vi "DAQtetris.vi"() -> ()   [LabVIEW 2018]
uses:
  <vilib>/Analysis/3filter.llb/Filter Passband Type.ctl
  <vilib>/Instr/_visa.llb/VISA Configure Serial Port (Instr).vi
  <vilib>/Analysis/3filter.llb/Butterworth Filter (DBL).vi
  <vilib>/Utility/file.llb/Write Delimited Spreadsheet (I64).vi
  <vilib>/Analysis/NI_AALBase.lvlib
panel:
  in  "Cancel Button":bool=TRUE
  out "error out":errorcluster
  out "stop 2":bool=TRUE
  in  "error in (no error)":errorcluster
  in  "Python version":string="3.6"
  out "AI2 2":i16(graph)
  out "AI1 2":i16(graph)
  out "AI0 2":i16(graph)
  in  "y 3":i16=8
  in  "y 2":i16=4
  in  "y":i16=7
  out "Up":bool
  out "Right":bool
  out "Left":bool
  in  "TR":dbl(slide)=2.5718194254445967e-05 scale=0.0..0.0001 scale format="%#_9g"
  in  "TT":dbl(slide)=2.633744855967078e-05 scale=0.0..0.0001 scale format="%#_9g"
  in  "TL":dbl(slide)=4.78796169630643e-05 scale=0.0..0.0001 scale format="%#_9g"
  in  "Rang 3":dbl(knob)=1000.0 scale=0.0..2000.0
  in  "Rang 2":dbl(knob)=1000.0 scale=0.0..2000.0
  in  "Rang 1":dbl(knob)=1000.0 scale=0.0..2000.0
  in  "File name":string="data111"
  in  "Record Button":bool
  out "Data Size":i32=4943
  out "Time left":u32
  in  "Time length(ms)":i32=100000
  in  "Timer":bool
  out "appended array":u16[][](array[numeric])
  out "Loop Time":u32
  in  "baud rate (9600)":u32=256000
  out "AI2":u16(graph)=19
  out "AI1":u16(graph)
  in  "Command":string="\u0000\u0000\u0006\u0004"
  in  "Disconnect":bool
  in  "Connect":bool
  out "AI0":u16(graph)=51
  in  "Send Command":bool
  in  "stop":bool
  out "read buffer":string
  in  "VISA resource name":refnum<visa-resource-name>="COM3"
  # "meDAQ v1.0\nXiangpeng"
  # "Wireless DAQ for Wearable Device"
  # "L"
  # "Display Scale"
  # "Initialization"
  # "Data Recording"
  # "T"
  # "Advanced Bluetooth Operation"
  # "R"
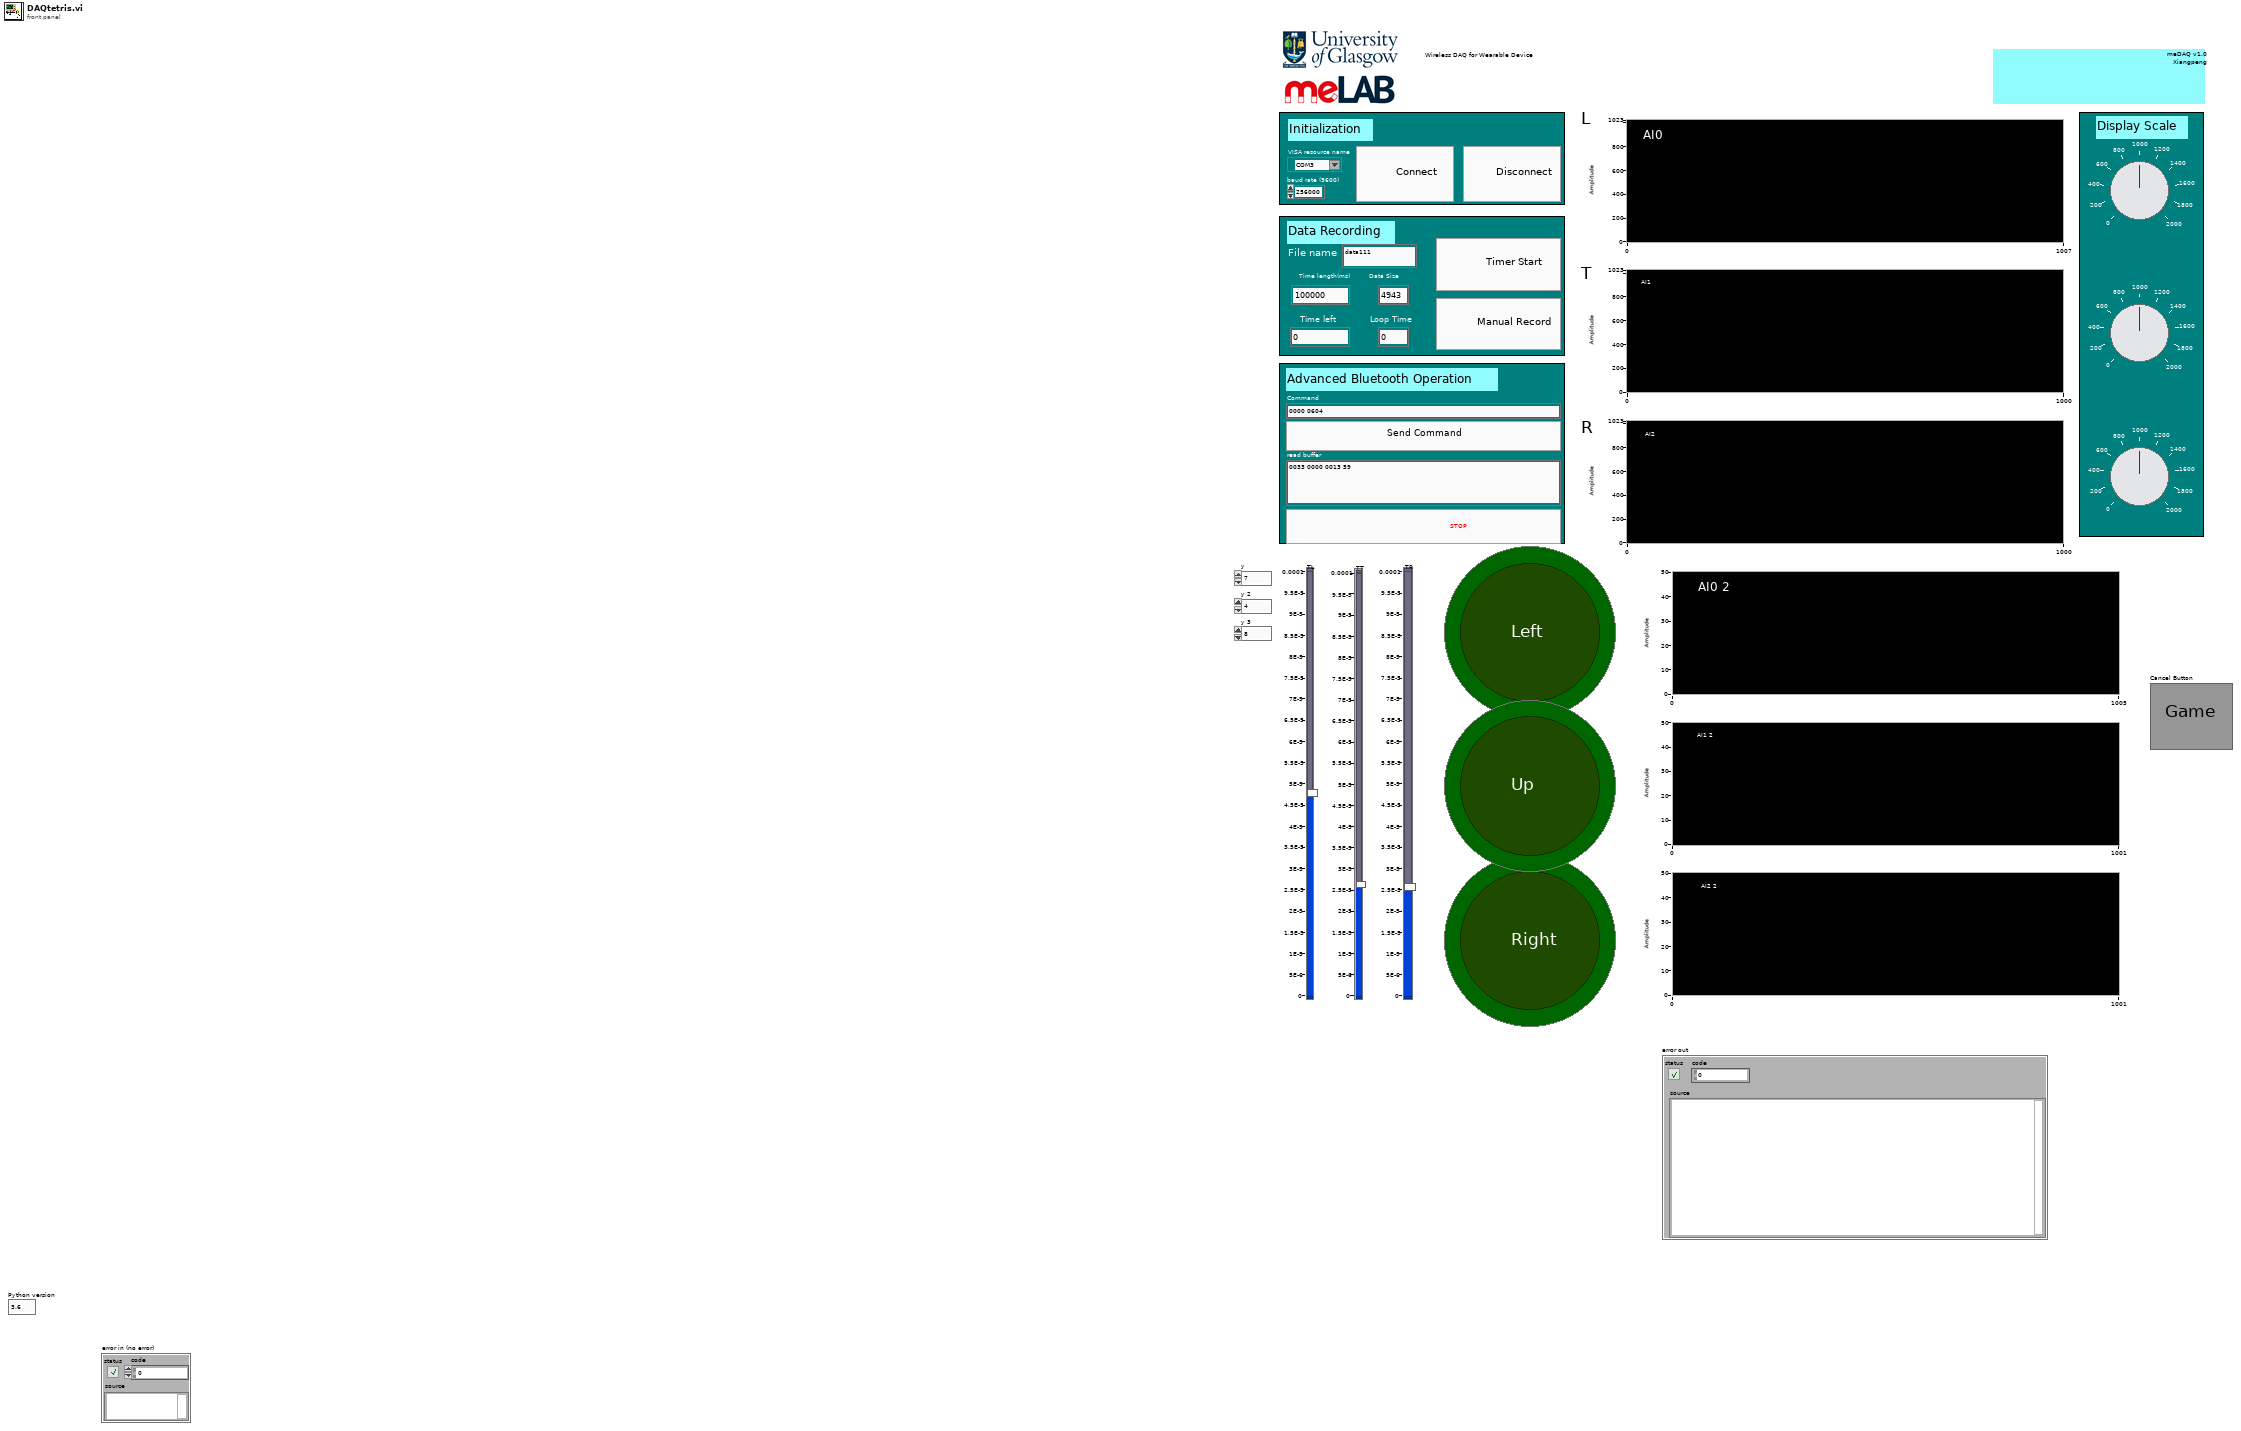
[diagram p1: front panel]
types:
  T1 = typedef "Sound Output Task ID.ctl" = u32
  T2 = typedef "NI_AALBase.lvlib/Filter Passband Type.ctl" = enum32{"Lowpass", "Highpass", "Bandpass", "Bandstop"}
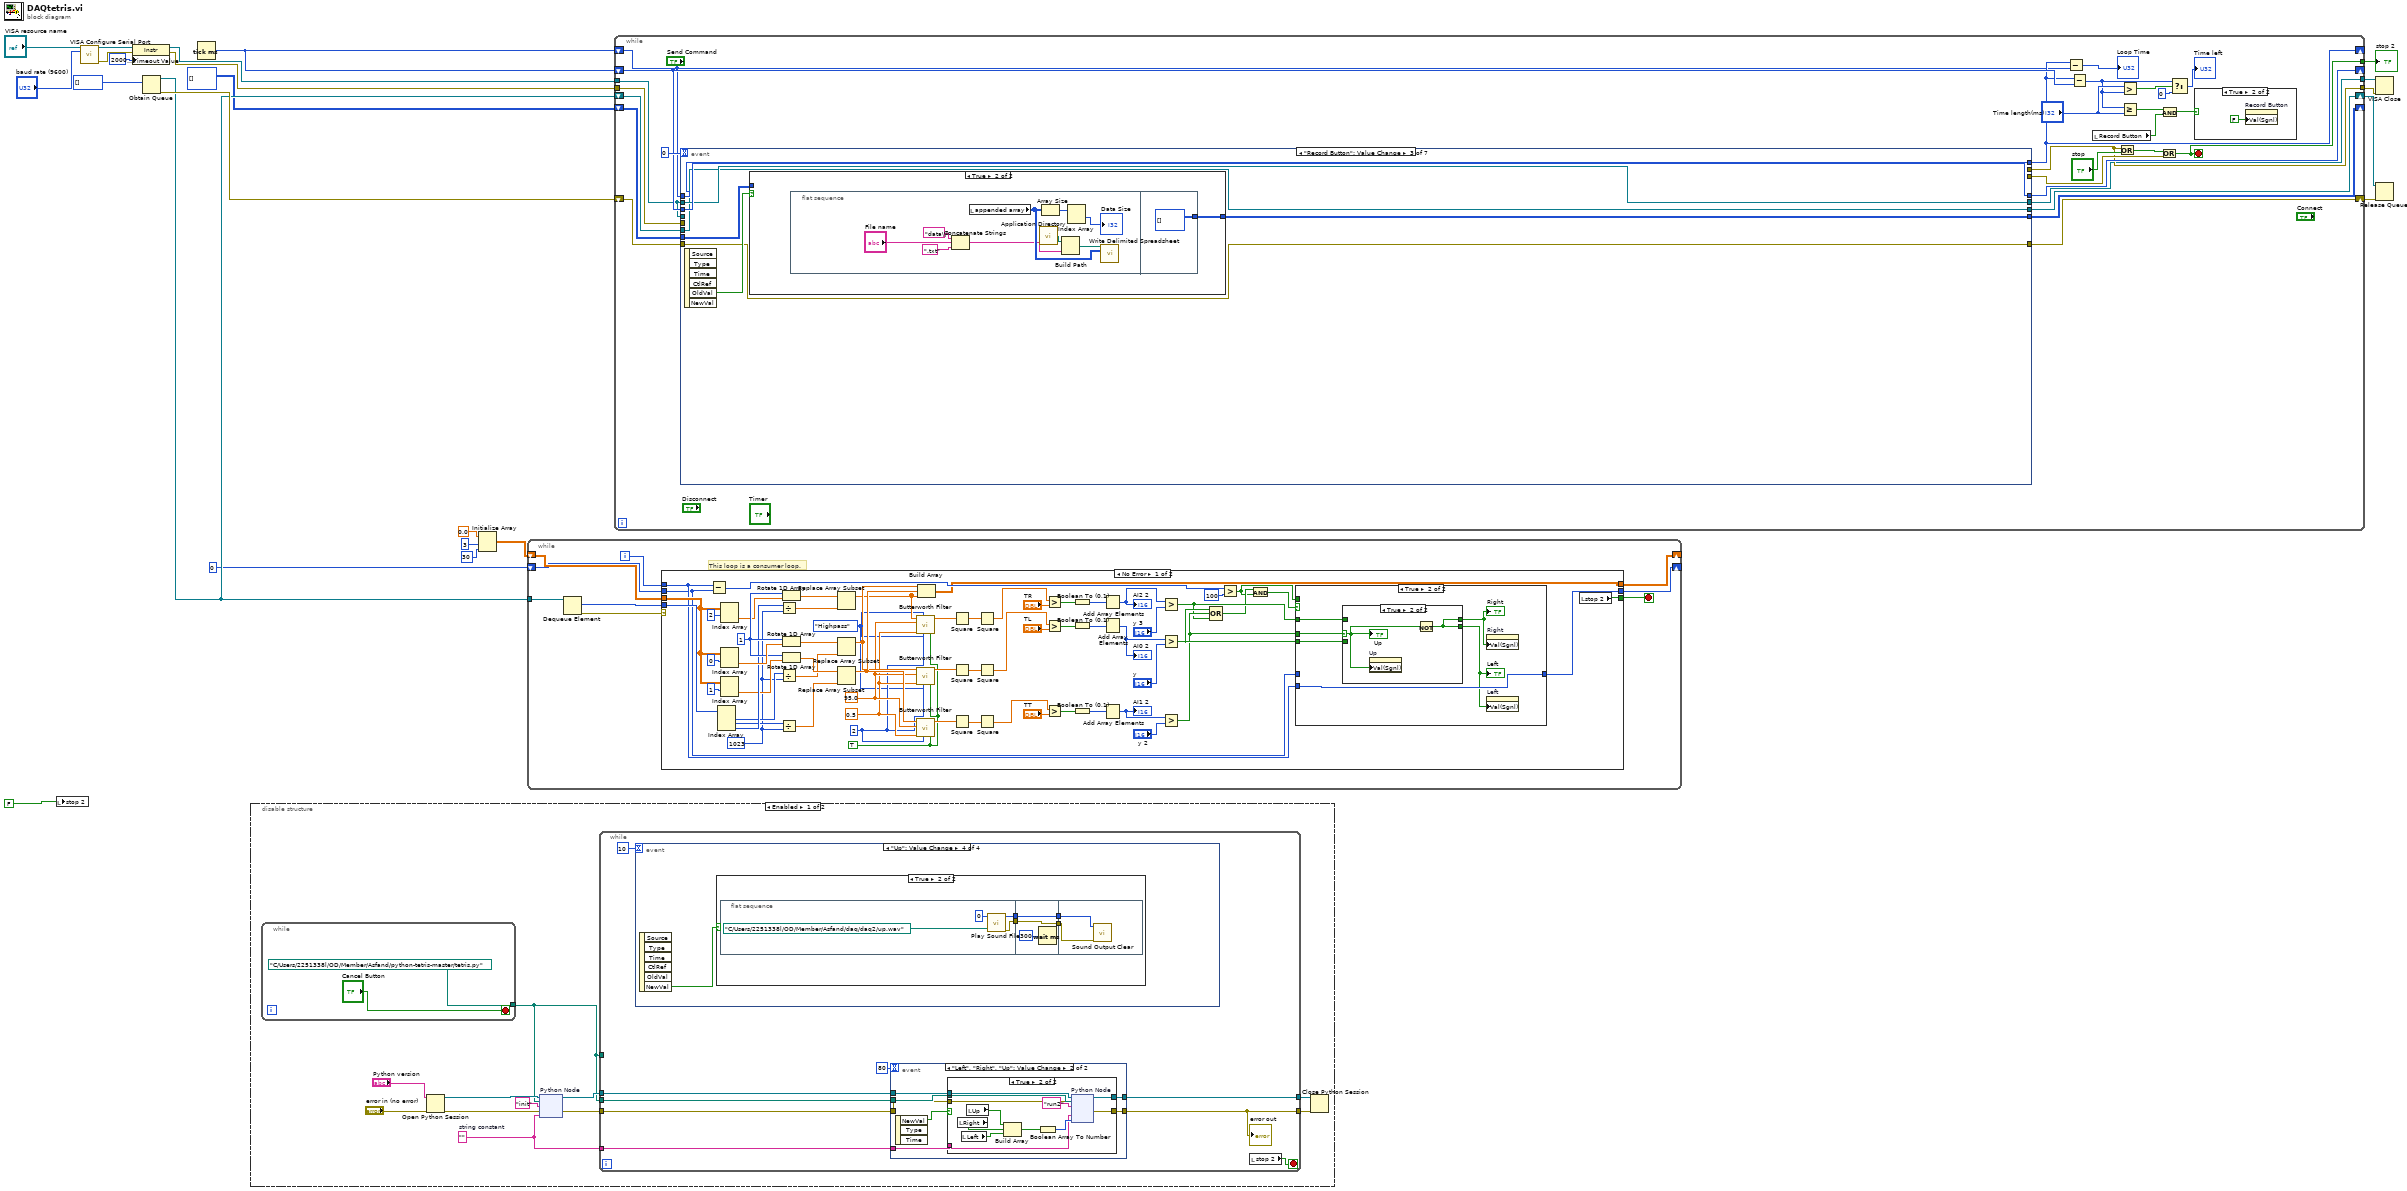
[diagram p0: block diagram]
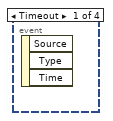
[diagram p2: hidden frame]
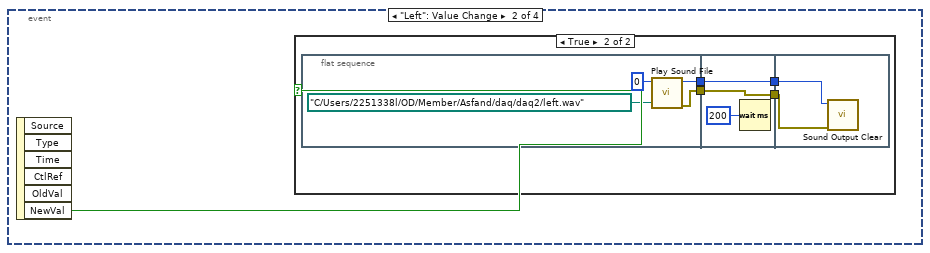
[diagram p3: hidden frame]
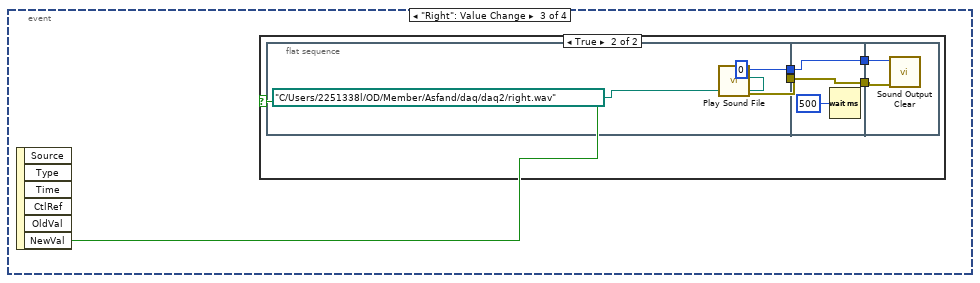
[diagram p5: hidden frame]
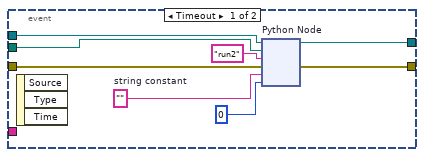
[diagram p8: hidden frame]
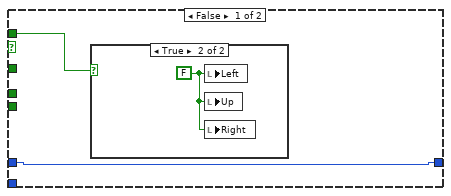
[diagram p11: hidden frame]
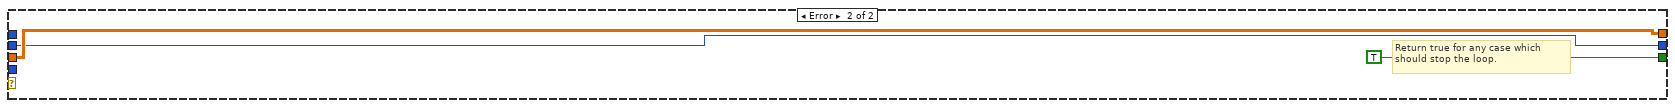
[diagram p14: hidden frame]
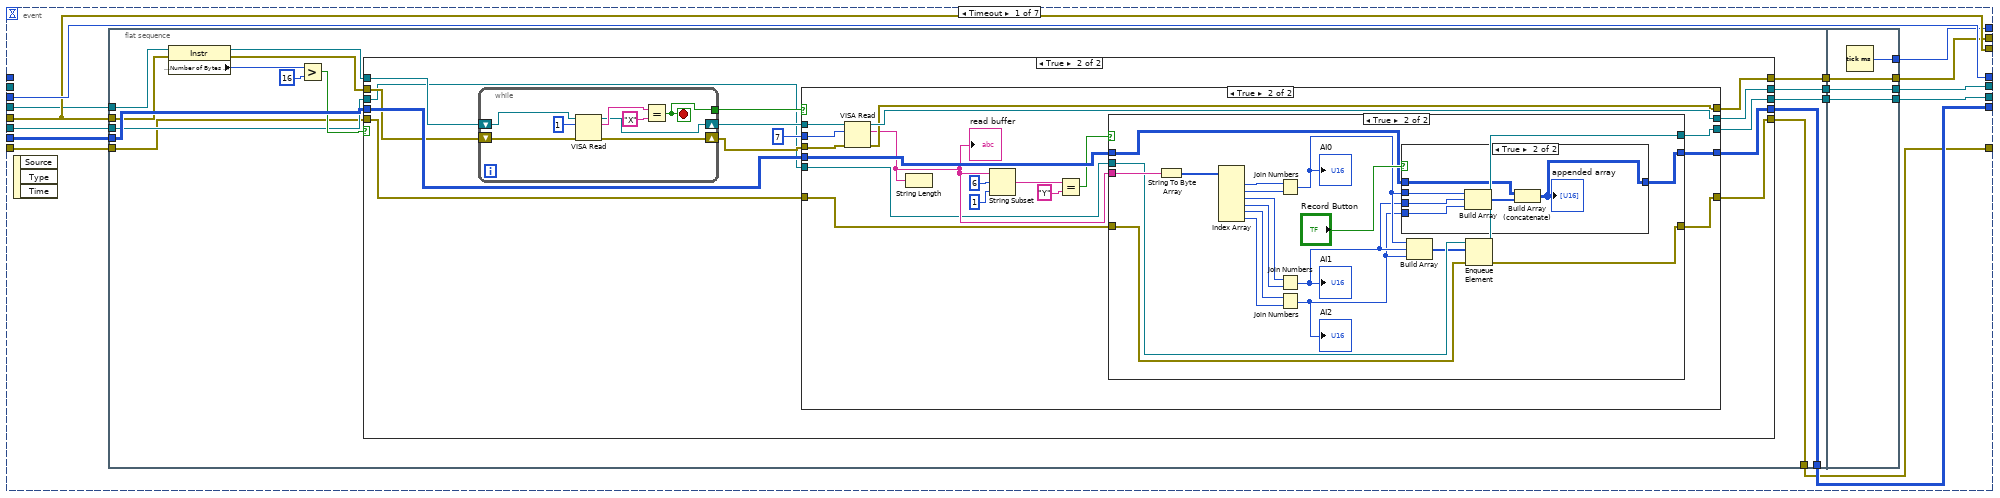
[diagram p16: hidden frame]
diagram:
  n1 = local write "stop 2"(FALSE ("stop 2")) -> ()
  n2 = call-poly "VISA Configure Serial Port"("VISA resource name"="VISA resource name", "baud rate (9600)"="baud rate (9600)") -> ("VISA resource name out"=w17:refnum<visa-resource-name>, "error out"=w16:errorcluster)  [unwired: 12 in]
  n3 = property class="Instr"(reference=w17, error in=w16, "General Settings:Timeout Value"=u32 2000) -> (reference out=w14:refnum<visa-resource-name>, error out=w15:errorcluster)
  n4 = Obtain Queue(element data type=u16[] []) -> (queue out=w10:refnum<queue>, error out=w13:errorcluster)  [unwired: 4 in, 1 out]
  n5 = Tick Count (ms)() -> (millisecond timer value=w19:u32)
  n6 = disable-structure shown="Enabled" {
    frame Enabled {
      w25 = ""  # string constant
      n7 = while {
        tunnel: [path "C:/Users/2251338l/OD/Member/Asfand/python-tetris-master/tetris.py" ("module path")] -> w24
        stop <- "Cancel Button" stop-if-true
      }
      n8 = Open Python Session(python version="Python version", 3:"error in (no error)") -> (session out=w31:refnum<k35>, error out=w30:errorcluster)  [unwired: 1 in]
      n9 = node "Python Node"(w31, w24, "init" ("function name"), w30, w25) -> (w27:refnum<k35>, w26:errorcluster)  [unwired: 1 in, 2 out]
      n10 = while {
        tunnel: [w37] -> w29
        tunnel: [w41] -> w28
        tunnel: w27 -> [w44]
        tunnel: w26 -> [w43]
        tunnel: w24 -> [w42]
        tunnel: w25 -> [w38]
        tunnel: w24 -> [_]
        stop <- w40 stop-if-true
        n11 = event shown="[3] \"Up\": Value Change" {
          selector: _ -> [_ _ _ _]
          dyn-events: _ -> [_ _ _ _]
          timeout: 10 -> [_ _ _ _]
          event Timeout {
            n12 = event-data() -> ()  [unwired: 1 in, 3 out]
          }
          event "Left": Value Change {
            n13 = event-data() -> ("NewVal"=w46:bool)  [unwired: 1 in, 5 out]
            n14 = case shown="True" w46 {
              frame False {
              }
              frame True {
                n15 = flat-sequence {
                  tunnel: [w54] -> w50
                  tunnel: [w51] -> w47
                  tunnel: w50 -> [w57]
                  tunnel: [w57] -> w49
                  tunnel: [w55] -> w48
                  tunnel: w47 -> [w55]
                  tunnel: w49 -> [w58]
                  tunnel: w48 -> [w59]
                  frame #0 {
                    n16 = call <vilib>:"Play Sound File.vi"("path"=path "C:/Users/2251338l/OD/Member/Asfand/daq/daq2/left.wav" ("Sound File Path"), "device ID"=u32 0) -> ("error out"=w51:errorcluster, "task ID"=w54:T1)  [unwired: 8 in]
                  }
                  frame #1 {
                    n17 = Wait (ms)(milliseconds to wait=u32 200) -> ()  [unwired: 1 out]
                  }
                  frame #2 {
                    n18 = call <vilib>:"Sound Output Clear.vi"("error in (no error)"=w59, "task ID"=w58) -> ()  [unwired: 9 in, 1 out]
                  }
                }
              }
            }
          }
          event "Right": Value Change {
            n19 = event-data() -> ("NewVal"=w60:bool)  [unwired: 1 in, 5 out]
            n20 = case shown="True" w60 {
              frame False {
              }
              frame True {
                n21 = flat-sequence {
                  tunnel: [w68] -> w64
                  tunnel: [w66] -> w63
                  tunnel: w64 -> [w69]
                  tunnel: [w70] -> w62
                  tunnel: w63 -> [w70]
                  tunnel: [w69] -> w61
                  tunnel: w62 -> [w73]
                  tunnel: w61 -> [w72]
                  frame #0 {
                    n22 = call <vilib>:"Play Sound File.vi"("path"=path "C:/Users/2251338l/OD/Member/Asfand/daq/daq2/right.wav" ("Sound File Path"), "device ID"=u32 0) -> ("error out"=w66:errorcluster, "task ID"=w68:T1)  [unwired: 8 in]
                  }
                  frame #1 {
                    n23 = Wait (ms)(milliseconds to wait=u32 500) -> ()  [unwired: 1 out]
                  }
                  frame #2 {
                    n24 = call <vilib>:"Sound Output Clear.vi"("error in (no error)"=w73, "task ID"=w72) -> ()  [unwired: 9 in, 1 out]
                  }
                }
              }
            }
          }
          event "Up": Value Change {
            n25 = event-data() -> ("NewVal"=w74:bool)  [unwired: 1 in, 5 out]
            n26 = case shown="True" w74 {
              frame False {
              }
              frame True {
                n27 = flat-sequence {
                  tunnel: [w82] -> w78
                  tunnel: [w80] -> w77
                  tunnel: w78 -> [w85]
                  tunnel: [w85] -> w76
                  tunnel: [w83] -> w75
                  tunnel: w77 -> [w83]
                  tunnel: w76 -> [w86]
                  tunnel: w75 -> [w87]
                  frame #0 {
                    n28 = call <vilib>:"Play Sound File.vi"("path"=path "C:/Users/2251338l/OD/Member/Asfand/daq/daq2/up.wav" ("Sound File Path"), "device ID"=u32 0) -> ("error out"=w80:errorcluster, "task ID"=w82:T1)  [unwired: 8 in]
                  }
                  frame #1 {
                    n29 = Wait (ms)(milliseconds to wait=u32 300) -> ()  [unwired: 1 out]
                  }
                  frame #2 {
                    n30 = call <vilib>:"Sound Output Clear.vi"("error in (no error)"=w87, "task ID"=w86) -> ()  [unwired: 9 in, 1 out]
                  }
                }
              }
            }
          }
        }
        n31 = event shown="[1] \"Left\", \"Right\", \"Up\": Value Change" {
          selector: _ -> [_ _]
          dyn-events: _ -> [_ _]
          timeout: 80 -> [_ _]
          tunnel: w44 -> [w95 w98]
          tunnel: w43 -> [w93 w99]
          tunnel: w42 -> [w91 w102]
          tunnel: [w90 w101] -> w37
          tunnel: [w89 w100] -> w41
          tunnel: w38 -> [_ w97]
          event Timeout {
            w92 = ""  # string constant
            n32 = event-data() -> ()  [unwired: 1 in, 3 out]
            n33 = node "Python Node"(w95, w91, "run2" ("function name"), w93, w92, u32 0 ("device ID")) -> (w90:refnum<k35>, w89:errorcluster)  [unwired: 2 in, 2 out]
          }
          event "Left", "Right", "Up": Value Change {
            n34 = event-data() -> ("NewVal"=w96:bool)  [unwired: 1 in, 2 out]
            n35 = case shown="True" w96 {
              tunnel: w102 -> [_ w111]
              tunnel: [w104 w109] -> w101
              tunnel: [w103 w108] -> w100
              tunnel: w99 -> [w103 w107]
              tunnel: w98 -> [w104 w106]
              tunnel: w97 -> [_ w105]
              frame False {
              }
              frame True {
                n36 = local read "Right"() -> (w114:bool)
                n37 = local read "Left"() -> (w113:bool)
                n38 = local read "Up"() -> (w115:bool)
                n39 = Build Array(w115, w114, w113) -> (w112:bool[])
                n40 = Boolean Array To Number(Boolean array=w112) -> (number=w116:u32)
                n41 = node "Python Node"(w106, w111, "run2" ("function name"), w107, w105, w116) -> (w109:refnum<k35>, w108:errorcluster)  [unwired: 2 in, 2 out]
              }
            }
          }
        }
        "error out" <- w41
        n42 = local read "stop 2"() -> (w40:bool)
      }
      n43 = Close Python Session(session in=w29, error in=w28) -> ()  [unwired: 1 out]
    }
    frame Disabled {
    }
  }
  n44 = Initialize Array(0.0, 3 ("dimension size"), 30 ("dimension size")) -> (w4:dbl[][])
  n45 = while {
    tunnel: w10 -> [w125]
    shift-right: [w120] -> _
    shift-left: w4 -> [w121]
    shift-right: [w119] -> _
    shift-left: 0 -> [w117]
    i -> [w118]
    stop <- w122 stop-if-true
    # "This loop is a consumer loop."
    n46 = Dequeue Element(queue=w125) -> (element=w123:u16[], error out=w124:errorcluster)  [unwired: 2 in, 2 out]
    n47 = case shown="No Error" w124 {
      tunnel: w123 -> [w187 _]
      tunnel: [w126 TRUE] -> w122
      tunnel: w121 -> [w181 w204]
      tunnel: [w138 w204] -> w120
      tunnel: [w146 w203] -> w119
      tunnel: w118 -> [w145 _]
      tunnel: w117 -> [w144 w203]
      frame No Error {
        w128 = TRUE ("init/cont (init:F)")
        w131 = 95.0 ("sampling freq: fs")
        w129 = 2 ("order")
        w130 = 0.5 ("low cutoff freq: fl")
        w127 = Filter_Passband_Type."Highpass" ("filter type")
        w157 = u16 1023 ("y")
        w186 = 1 ("n")
        n48 = Subtract(x=w145, y=w144) -> (x-y=w143:i32)
        n49 = Index Array(array=w187) -> (element #1=w161:u16, element #2=w182:u16, element #3=w183:u16)  [unwired: 3 in]
        n50 = Index Array(array=w181, index (row)=2 ("index (col)")) -> (element=w179:dbl[])  [unwired: 1 in]
        n51 = Index Array(array=w181, index (row)=0 ("disabled index (col)")) -> (element=w189:dbl[])  [unwired: 1 in]
        n52 = Index Array(array=w181, index (row)=1 ("index (col)")) -> (element=w180:dbl[])  [unwired: 1 in]
        n53 = Divide(x=w183, y=w157) -> (x/y=w158:dbl)
        n54 = Divide(x=w161, y=w157) -> (x/y=w160:dbl)
        n55 = Divide(x=w182, y=w157) -> (x/y=w159:dbl)
        n56 = Rotate 1D Array(1:w179, 2:w186) -> (0:w184:dbl[])
        n57 = Rotate 1D Array(1:w189, 2:w186) -> (0:w188:dbl[])
        n58 = Rotate 1D Array(1:w180, 2:w186) -> (0:w185:dbl[])
        n59 = Replace Array Subset(array=w184, new element=w158) -> (w133:dbl[])  [unwired: 1 in]
        n60 = Replace Array Subset(array=w188, new element=w160) -> (w135:dbl[])  [unwired: 1 in]
        n61 = Replace Array Subset(array=w185, new element=w159) -> (w137:dbl[])  [unwired: 1 in]
        n62 = call-poly <vilib>:"Butterworth Filter.vi"("init/cont (init:F)"=w128, "order"=w129, "filter type"=w127, "low cutoff freq: fl"=w130, "sampling freq: fs"=w131, "X"=w133) -> ("Filtered X"=w132:dbl[])  [unwired: 2 in, 1 out]
        n63 = call-poly <vilib>:"Butterworth Filter.vi"("init/cont (init:F)"=w128, "order"=w129, "filter type"=w127, "low cutoff freq: fl"=w130, "sampling freq: fs"=w131, "X"=w135) -> ("Filtered X"=w134:dbl[])  [unwired: 2 in, 1 out]
        n64 = call-poly <vilib>:"Butterworth Filter.vi"("init/cont (init:F)"=w128, "order"=w129, "filter type"=w127, "low cutoff freq: fl"=w130, "sampling freq: fs"=w131, "X"=w137) -> ("Filtered X"=w136:dbl[])  [unwired: 2 in, 1 out]
        n65 = Build Array(w135, w137, w133) -> (w138:dbl[][])
        n66 = Square(x=w132) -> (x^2=w156:dbl[])
        n67 = Square(x=w134) -> (x^2=w154:dbl[])
        n68 = Square(x=w136) -> (x^2=w155:dbl[])
        n69 = Square(x=w156) -> (x^2=w171:dbl[])
        n70 = Square(x=w154) -> (x^2=w175:dbl[])
        n71 = Square(x=w155) -> (x^2=w170:dbl[])
        n72 = Greater?(x=w171, y="TR") -> (0:w162:bool[])
        n73 = Greater?(x=w175, y="TL") -> (0:w169:bool[])
        n74 = Greater?(x=w170, y="TT") -> (0:w165:bool[])
        n75 = Boolean To (0,1)(Boolean=w162) -> (0, 1=w164:i16[])
        n76 = Boolean To (0,1)(Boolean=w169) -> (0, 1=w168:i16[])
        n77 = Boolean To (0,1)(Boolean=w165) -> (0, 1=w166:i16[])
        n78 = Add Array Elements(numeric array=w164) -> (sum=w153:i16)
        "AI2 2" <- w153
        n79 = Add Array Elements(numeric array=w168) -> (sum=w151:i16)
        "AI0 2" <- w151
        n80 = Add Array Elements(numeric array=w166) -> (sum=w152:i16)
        "AI1 2" <- w152
        n81 = Greater?(x=w153, y="y 3") -> (0:w148:bool)
        n82 = Greater?(x=w151, y="y") -> (0:w150:bool)
        n83 = Greater?(x=w152, y="y 2") -> (0:w149:bool)
        n84 = Compound Arithmetic op=OR(w150, w149, w148) -> (w141:bool)
        n85 = Greater?(x=w143, y=100) -> (0:w139:bool)
        n86 = And(x=w141, y=w139) -> (x .and. y?=w140:bool)
        n87 = case shown="True" w140 {
          tunnel: w150 -> [_ w195]
          tunnel: w149 -> [_ w197]
          tunnel: w148 -> [_ w196]
          tunnel: [w191 w198] -> w146
          tunnel: w145 -> [_ w198]
          tunnel: w144 -> [w191 _]
          tunnel: w139 -> [w190 _]
          frame False {
            n88 = case shown="True" w190 {
              frame False {
              }
              frame True {
                w192 = FALSE
                n89 = local write "Left"(w192) -> ()
                n90 = local write "Up"(w192) -> ()
                n91 = local write "Right"(w192) -> ()
              }
            }
          }
          frame True {
            n92 = case shown="True" w197 {
              selector: w197 -> [_ w201]
              tunnel: [w200 w202] -> w193
              tunnel: [w199 w202] -> w194
              tunnel: w196 -> [w200 _]
              tunnel: w195 -> [w199 _]
              frame False {
              }
              frame True {
                n93 = property on="Up" class="Bool (strict)"("Val(Sgnl)"=w201) -> ()  [unwired: 2 in, 2 out]
                n94 = Not(x=w201) -> (.not. x?=w202:bool)
                "Up" <- w201
              }
            }
            "Left" <- w194
            "Right" <- w193
            n95 = property on="Right" class="Bool (strict)"("Val(Sgnl)"=w193) -> ()  [unwired: 2 in, 2 out]
            n96 = property on="Left" class="Bool (strict)"("Val(Sgnl)"=w194) -> ()  [unwired: 2 in, 2 out]
          }
        }
        n97 = local read "stop 2"() -> (w126:bool)
      }
      frame Error {
        # "Return true for any case which should stop the loop."
      }
    }
  }
  n98 = while {
    tunnel: w14 -> [w216]
    tunnel: w15 -> [w231]
    tunnel: [w213] -> w22
    tunnel: [w214] -> w21
    shift-right: [w212] -> _
    shift-left: w19 -> [w211]
    shift-right: [w227] -> _
    shift-left: u16[][] [] ("appended array 2") -> [w215]
    shift-right: [w226] -> _
    shift-left: w19 -> [w225]
    shift-right: [w208] -> w12
    shift-left: w10 -> [w210]
    shift-right: [w207] -> w11
    shift-left: w13 -> [w209]
    tunnel: [w206] -> w3
    stop <- w206 stop-if-true
    n99 = event shown="[2] \"Record Button\": Value Change" {
      selector: _ -> [_ _ _ _ _ _ _]
      dyn-events: _ -> [_ _ _ _ _ _ _]
      timeout: 0 -> [_ _ _ _ _ _ _]
      tunnel: w216 -> [_ _ w366 w390 _ w404 w416]
      tunnel: w231 -> [w246 w355 _ w389 _ w405 w415]
      tunnel: [w246 _ _ w388 _ w403 w414] -> w229
      tunnel: [w243 w358 w369 w386 w395 w401 w410] -> w227
      tunnel: [w249 w356 w368 w387 w396 w402 w411] -> w226
      tunnel: w225 -> [w249 w356 w368 w387 _ w402 w411]
      tunnel: w216 -> [w245 w359 _ _ _ _ _]
      tunnel: w215 -> [w244 w358 w367 w386 w395 w401 w410]
      tunnel: [w242 w355 _ _ _ _ _] -> w214
      tunnel: [w241 w359 w366 _ _ _ _] -> w213
      tunnel: [w240 w357 w365 w385 w394 w400 w409] -> w212
      tunnel: w211 -> [_ w357 w365 w385 w394 w400 w409]
      tunnel: w210 -> [w239 w348 w364 w384 w393 w399 w408]
      tunnel: w209 -> [w238 w347 w363 w383 w392 w398 w407]
      tunnel: [w236 w348 w364 w384 w393 w399 w408] -> w208
      tunnel: [w235 w347 w363 w383 w392 w398 w407] -> w207
      event Timeout {
        n100 = event-data() -> ()  [unwired: 1 in, 3 out]
        n101 = flat-sequence {
          tunnel: [w264] -> w248
          tunnel: [w263] -> w247
          tunnel: [w262] -> w243
          tunnel: w244 -> [w261]
          tunnel: w245 -> [w260]
          tunnel: w246 -> [w258]
          tunnel: w239 -> [w253]
          tunnel: w238 -> [w252]
          tunnel: [w251] -> w237
          tunnel: [w250] -> w235
          tunnel: [w345] -> w242
          tunnel: [w346] -> w241
          tunnel: w248 -> [w346]
          tunnel: w247 -> [w345]
          tunnel: [w344] -> w240
          tunnel: w237 -> [w343]
          tunnel: [w343] -> w236
          frame #0 {
            n102 = property class="Instr"(reference=w260, error in=w258) -> (reference out=w259:refnum<visa-resource-name>, error out=w257:errorcluster, "Serial Settings:Number of Bytes at Serial Port"=w255:u32)
            n103 = Greater?(x=w255, y=u32 16) -> (0:w256:bool)
            n104 = case shown="True" w256 {
              tunnel: [w269 w283] -> w264
              tunnel: [w268 w282] -> w263
              tunnel: [w267 w280] -> w262
              tunnel: w261 -> [w267 w279]
              tunnel: w259 -> [w269 w278]
              tunnel: w257 -> [w268 w277]
              tunnel: w253 -> [w266 w273]
              tunnel: w252 -> [w265 w272]
              tunnel: [w266 w271] -> w251
              tunnel: [w265 w270] -> w250
              frame False {
              }
              frame True {
                n105 = while {
                  tunnel: [w284] -> w274
                  shift-right: [w286] -> w276
                  shift-left: w278 -> [w291]
                  shift-right: [w285] -> w275
                  shift-left: w277 -> [w289]
                  stop <- w284 stop-if-true
                  n106 = VISA Read(VISA resource name=w291, byte count=u32 1, error in (no error)=w289) -> (VISA resource name out=w286:refnum<visa-resource-name>, read buffer=w287:string, error out=w285:errorcluster)  [unwired: 1 out]
                  n107 = Equal?(x=w287, y="X" ("substring")) -> (x = y?=w284:bool)
                }
                n108 = case shown="True" w274 {
                  tunnel: w276 -> [w295 w301]
                  tunnel: [w295 w313] -> w283
                  tunnel: [w294 w312] -> w282
                  tunnel: u32 7 ("Serial Settings:Number of Bytes at Serial Port") -> [_ w307]
                  tunnel: [w296 w306] -> w280
                  tunnel: w279 -> [w296 w305]
                  tunnel: w275 -> [w294 w304]
                  tunnel: w273 -> [w292 w300]
                  tunnel: w272 -> [w293 w299]
                  tunnel: [w292 w298] -> w271
                  tunnel: [w293 w297] -> w270
                  frame False {
                  }
                  frame True {
                    n109 = VISA Read(VISA resource name=w301, byte count=w307, error in (no error)=w304) -> (VISA resource name out=w313:refnum<visa-resource-name>, read buffer=w302:string, error out=w312:errorcluster)  [unwired: 1 out]
                    "read buffer" <- w302
                    n110 = String Length(string=w302) -> ()  [unwired: 1 out]
                    n111 = String Subset(string=w302, offset (0)=6, length (rest)=1 ("length (rest)")) -> (substring=w309:string)
                    n112 = Equal?(x=w309, y="Y" ("substring")) -> (x = y?=w303:bool)
                    n113 = case shown="True" w303 {
                      tunnel: w302 -> [_ w334]
                      tunnel: [w316 w326] -> w306
                      tunnel: w305 -> [w316 w325]
                      tunnel: w300 -> [w315 w324]
                      tunnel: w299 -> [w314 w323]
                      tunnel: [w315 w322] -> w298
                      tunnel: [w314 w321] -> w297
                      frame False {
                      }
                      frame True {
                        n114 = String To Byte Array(string=w334) -> (unsigned byte array=w335:u8[])
                        n115 = Index Array(array=w335) -> (element #1=w333:u8, element #2=w332:u8, element #3=w331:u8, element #4=w330:u8, element #5=w329:u8, element #6=w328:u8)  [unwired: 6 in]
                        n116 = Join Numbers(hi=w333, lo=w332) -> ((hi.lo)=w320:u16)
                        "AI0" <- w320
                        n117 = Join Numbers(hi=w331, lo=w330) -> ((hi.lo)=w319:u16)
                        "AI1" <- w319
                        n118 = Join Numbers(hi=w329, lo=w328) -> ((hi.lo)=w318:u16)
                        "AI2" <- w318
                        n119 = case shown="True" "Record Button" {
                          tunnel: w320 -> [_ w342]
                          tunnel: w319 -> [_ w341]
                          tunnel: w318 -> [_ w340]
                          tunnel: [w336 w337] -> w326
                          tunnel: w325 -> [w336 w338]
                          frame False {
                          }
                          frame True {
                            n120 = Build Array(w342, w341, w340) -> (w339:u16[])
                            n121 = Build Array (concatenate)(w338, w339) -> (w337:u16[][])
                            "appended array" <- w337
                          }
                        }
                        n122 = Build Array(w320, w319, w318) -> (w317:u16[])
                        n123 = Enqueue Element(queue=w324, element=w317, error in (no error)=w323) -> (queue out=w322:refnum<queue>, error out=w321:errorcluster)  [unwired: 1 in, 1 out]
                      }
                    }
                  }
                }
              }
            }
          }
          frame #1 {
            n124 = Tick Count (ms)() -> (millisecond timer value=w344:u32)
          }
        }
      }
      event "Rang 1", "Rang 3", "Rang 2": Value Change {
        n125 = event-data() -> ()  [unwired: 1 in, 6 out]
        n126 = property on="AI1" class="WFChart (strict)"() -> ("XScale.Maximum"=w352:dbl)  [unwired: 2 in, 2 out]
        n127 = property on="AI0" class="WFChart (strict)"() -> ("XScale.Maximum"=w360:dbl)  [unwired: 2 in, 2 out]
        n128 = property on="AI2" class="WFChart (strict)"() -> ("XScale.Maximum"=w350:dbl)  [unwired: 2 in, 2 out]
        n129 = Subtract(x=w352, y="Rang 2") -> (x-y=w351:dbl)
        n130 = Subtract(x=w360, y="Rang 1") -> (x-y=w362:dbl)
        n131 = Subtract(x=w350, y="Rang 3") -> (x-y=w349:dbl)
        n132 = property on="AI1" class="WFChart (strict)"("XScale.Minimum"=w351) -> ()  [unwired: 2 in, 2 out]
        n133 = property on="AI0" class="WFChart (strict)"("XScale.Minimum"=w362) -> ()  [unwired: 2 in, 2 out]
        n134 = property on="AI2" class="WFChart (strict)"("XScale.Minimum"=w349) -> ()  [unwired: 2 in, 2 out]
      }
      event "Record Button": Value Change {
        n135 = event-data() -> ("OldVal"=w370:bool)  [unwired: 1 in, 5 out]
        n136 = case shown="True" w370 {
          tunnel: [w371 w372] -> w369
          tunnel: w367 -> [w371 _]
          frame False {
          }
          frame True {
            n137 = flat-sequence {
              tunnel: [u16[][] [] ("appended array 2")] -> w372
              frame #0 {
                n138 = Concatenate Strings("data\\" ("name or relative path"), "File name", ".txt" ("string")) -> (w375:string)
                n139 = local read "appended array"() -> (w379:u16[][])
                n140 = call <vilib>:"Application Directory.vi"() -> ("Application Directory"=w373:path)
                n141 = Array Size(array=w379) -> (size(s)=w381:i32[])
                n142 = Build Path(base path=w373, name or relative path=w375) -> (appended path=w374:path)
                n143 = Index Array(array=w381) -> (element #1=→"Data Size":i32)  [unwired: 2 in, 1 out]
                n144 = call-poly <vilib>:"Write Delimited Spreadsheet.vi"("file path (dialog if empty)"=w374, "2D data"=w379) -> ()  [unwired: 12 in, 2 out]
              }
              frame #1 {
              }
            }
          }
        }
      }
      event "Send Command": Value Change {
        n145 = event-data() -> ()  [unwired: 1 in, 6 out]
        n146 = VISA Write(VISA resource name=w390, write buffer="Command", error in (no error)=w389) -> (error out=w388:errorcluster)  [unwired: 2 out]
      }
      event "Timer": Value Change {
        n147 = event-data() -> ()  [unwired: 1 in, 6 out]
        n148 = local write "Record Button"(TRUE ("Record Button")) -> ()
        n149 = Tick Count (ms)() -> (millisecond timer value=w396:u32)
      }
      event "Disconnect": Value Change {
        n150 = event-data() -> ()  [unwired: 1 in, 6 out]
        n151 = VISA Write(VISA resource name=w404, write buffer="\u0000\u0001\u0003\u0000\u0000" ("write buffer 2"), error in (no error)=w405) -> (error out=w403:errorcluster)  [unwired: 2 out]
      }
      event "Connect": Value Change {
        n152 = event-data() -> ()  [unwired: 1 in, 6 out]
        n153 = flat-sequence {
          tunnel: [w432] -> w427
          tunnel: [w431] -> w426
          tunnel: w416 -> [w430]
          tunnel: w415 -> [w429]
          tunnel: [w428] -> w425
          tunnel: [w437] -> w424
          tunnel: w427 -> [w440]
          tunnel: [w440] -> w423
          tunnel: w426 -> [w437]
          tunnel: w425 -> [w438]
          tunnel: [w445] -> w422
          tunnel: [w444] -> w421
          tunnel: w424 -> [w449]
          tunnel: w423 -> [w448]
          tunnel: [w443] -> w420
          tunnel: w422 -> [w452]
          tunnel: w421 -> [w451]
          tunnel: [w452] -> w419
          tunnel: [w451] -> w418
          tunnel: w420 -> [w450]
          tunnel: [w450] -> w417
          tunnel: w419 -> [w456]
          tunnel: w418 -> [w455]
          tunnel: w417 -> [w454]
          tunnel: [w458] -> w413
          tunnel: [w457] -> w412
          tunnel: [w459] -> w414
          tunnel: w413 -> [w461]
          tunnel: w412 -> [w460]
          frame #0 {
            n154 = VISA Write(VISA resource name=w430, write buffer="\u0000\u0001\u0003\u0000\u0002" ("write buffer 2"), error in (no error)=w429) -> (VISA resource name out=w436:refnum<visa-resource-name>, error out=w433:errorcluster)  [unwired: 1 out]
            n155 = VISA Write(VISA resource name=w436, write buffer="\u0000\u0001\u0003\u0000\u0000" ("write buffer 2"), error in (no error)=w433) -> (VISA resource name out=w431:refnum<visa-resource-name>, return count=w428:u32, error out=w432:errorcluster)
          }
          frame #1 {
            n156 = VISA Read(VISA resource name=w437, byte count=w438) -> ()  [unwired: 1 in, 4 out]
            n157 = Wait (ms)(milliseconds to wait=u32 10) -> ()  [unwired: 1 out]
          }
          frame #2 {
            (unwired) "\u0000\u000f\u0006\u0003šIF·²\f\u0000\u0006\u0000\u0016\u0000d\u0000\u0000\u0000" ("write buffer")
            (unwired) "\u0000\u000f\u0006\u0003(WF凡\f\u0000\u0006\u0000\u0016\u0000d\u0000\u0000\u0000" ("write buffer")
            (unwired) "\u0000\u000f\u0006\u0003ß\u0013±«^ô\u0000\u0006\u0000\u0016\u0000d\u0000\u0000\u0000" ("write buffer")
            n158 = Select(t="\u0000\u000f\u0006\u0003¶x\u0005s\u0004x\u0000\u0006\u0000\u0016\u0000d\u0000\u0000\u0000" ("write buffer"), s=TRUE, f="\u0000\u000f\u0006\u0003ß\u0013±«^ô\u0000<\u0000L\u0000d\u0000\u0000\u0000" ("write buffer")) -> (s? t:f=w446:string)
            n159 = VISA Write(VISA resource name=w449, write buffer=w446, error in (no error)=w448) -> (VISA resource name out=w445:refnum<visa-resource-name>, return count=w443:u32, error out=w444:errorcluster)
          }
          frame #3 {
            n160 = Wait (ms)(milliseconds to wait=u32 10) -> ()  [unwired: 1 out]
          }
          frame #4 {
            n161 = VISA Read(VISA resource name=w456, byte count=w454, error in (no error)=w455) -> (VISA resource name out=w458:refnum<visa-resource-name>, error out=w457:errorcluster)  [unwired: 2 out]
          }
          frame #5 {
            n162 = VISA Write(VISA resource name=w461, write buffer="\u0000\t\u0003\u0002\u0000\u0006\u0000\u0017\u0000\u0000\u0000(\u0000", error in (no error)=w460) -> (error out=w459:errorcluster)  [unwired: 2 out]
          }
        }
      }
    }
    n163 = Subtract(x=w212, y=w211) -> (x-y=→"Loop Time":u32)
    n164 = Subtract(x=w212, y=w225) -> (x-y=w219:u32)
    n165 = local read "Record Button"() -> (w224:bool)
    n166 = Or(x=w214, y="stop") -> (x .or. y?=w230:bool)
    n167 = Greater?(x="Time length(ms)", y=w219) -> (0:w220:bool)
    n168 = Greater Or Equal?(x=w219, y="Time length(ms)") -> (x >= y?=w223:bool)
    n169 = Or(x=w230, y=w229) -> (x .or. y?=w206:bool)
    n170 = And(x=w223, y=w224) -> (x .and. y?=w222:bool)
    n171 = Select(t=w219, s=w220, f=u32 0) -> (s? t:f=→"Time left":u32)
    n172 = case shown="True" w222 {
      frame False {
      }
      frame True {
        n173 = property on="Record Button" class="Bool (strict)"("Val(Sgnl)"=FALSE ("Record Button")) -> ()  [unwired: 2 in, 2 out]
      }
    }
  }
  "stop 2" <- w3
  n174 = VISA Close(VISA resource name=w22, error in (no error)=w21) -> ()  [unwired: 1 out]
  n175 = Release Queue(queue=w12, error in (no error)=w11) -> ()  [unwired: 1 in, 3 out]
